vi "date to day of the week.vi"(8 "error in (no error)":errorcluster, 9 "Day":u32, 10 "Month":T2, 11 "Year":u32) -> (0 "error out":errorcluster, 1 "no. of full weeks since 1 Jan 1900":u32, 2 "no. of days since 1 Jan 1900":u32, 3 "Day of the week":T1)   [LabVIEW 2021, in "Project Euler.lvlib"]
uses:
  Project Euler.lvlib
  months_of_the_year enum.ctl
  days_of_the_week enum.ctl
panel:
  out "no. of days in full months in current year":u32
  out "no. of days in current year":u32
  out "full years since 1 Jan 1900":u32[](array[numeric])
  out "no. of days in full years since 1 Jan 1900":u32
  out "no. of full years since 1 Jan 1900":u32
  # "Development\ncontrols/indicators useful for development and testing, but which are not outputs of the VI"
  # "Input\nInputs to the VI"
  # "Output\nOutputs of the VI"
  # "Description\n\nBlank VI with error handling case. \n\nSummarize the use of this VI in this space."
  # "This VI passed this test vector:\nsource = Windows 10 calendar\n1 Jan 1920 = Thursday\n1 Jan 1921 = Saturday\n27 May 1966 = Friday\n30 June 1966 = Thursday\n3 May 1992 = Sunday"
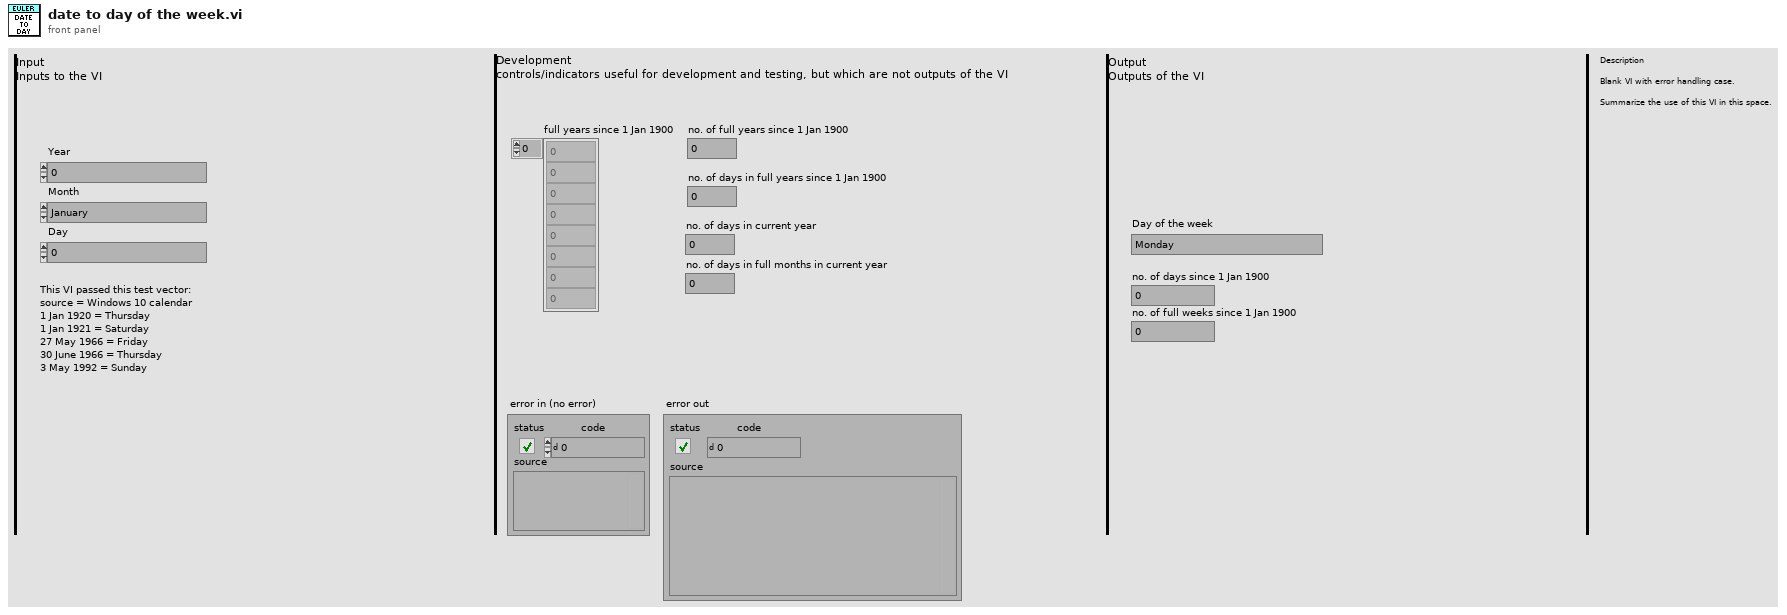
[diagram p1: front panel]
types:
  T1 = typedef "Project Euler.lvlib/days_of_the_week enum.ctl" = enum16{"Monday", "Tuesday", "Wednesday", "Thursday", "Friday", "Saturday", "Sunday"}
  T2 = typedef "Project Euler.lvlib/months_of_the_year enum.ctl" = enum16{"January", "February", "March", "April", "May", "June", "July", "August", "September", "October", "November", "December"}
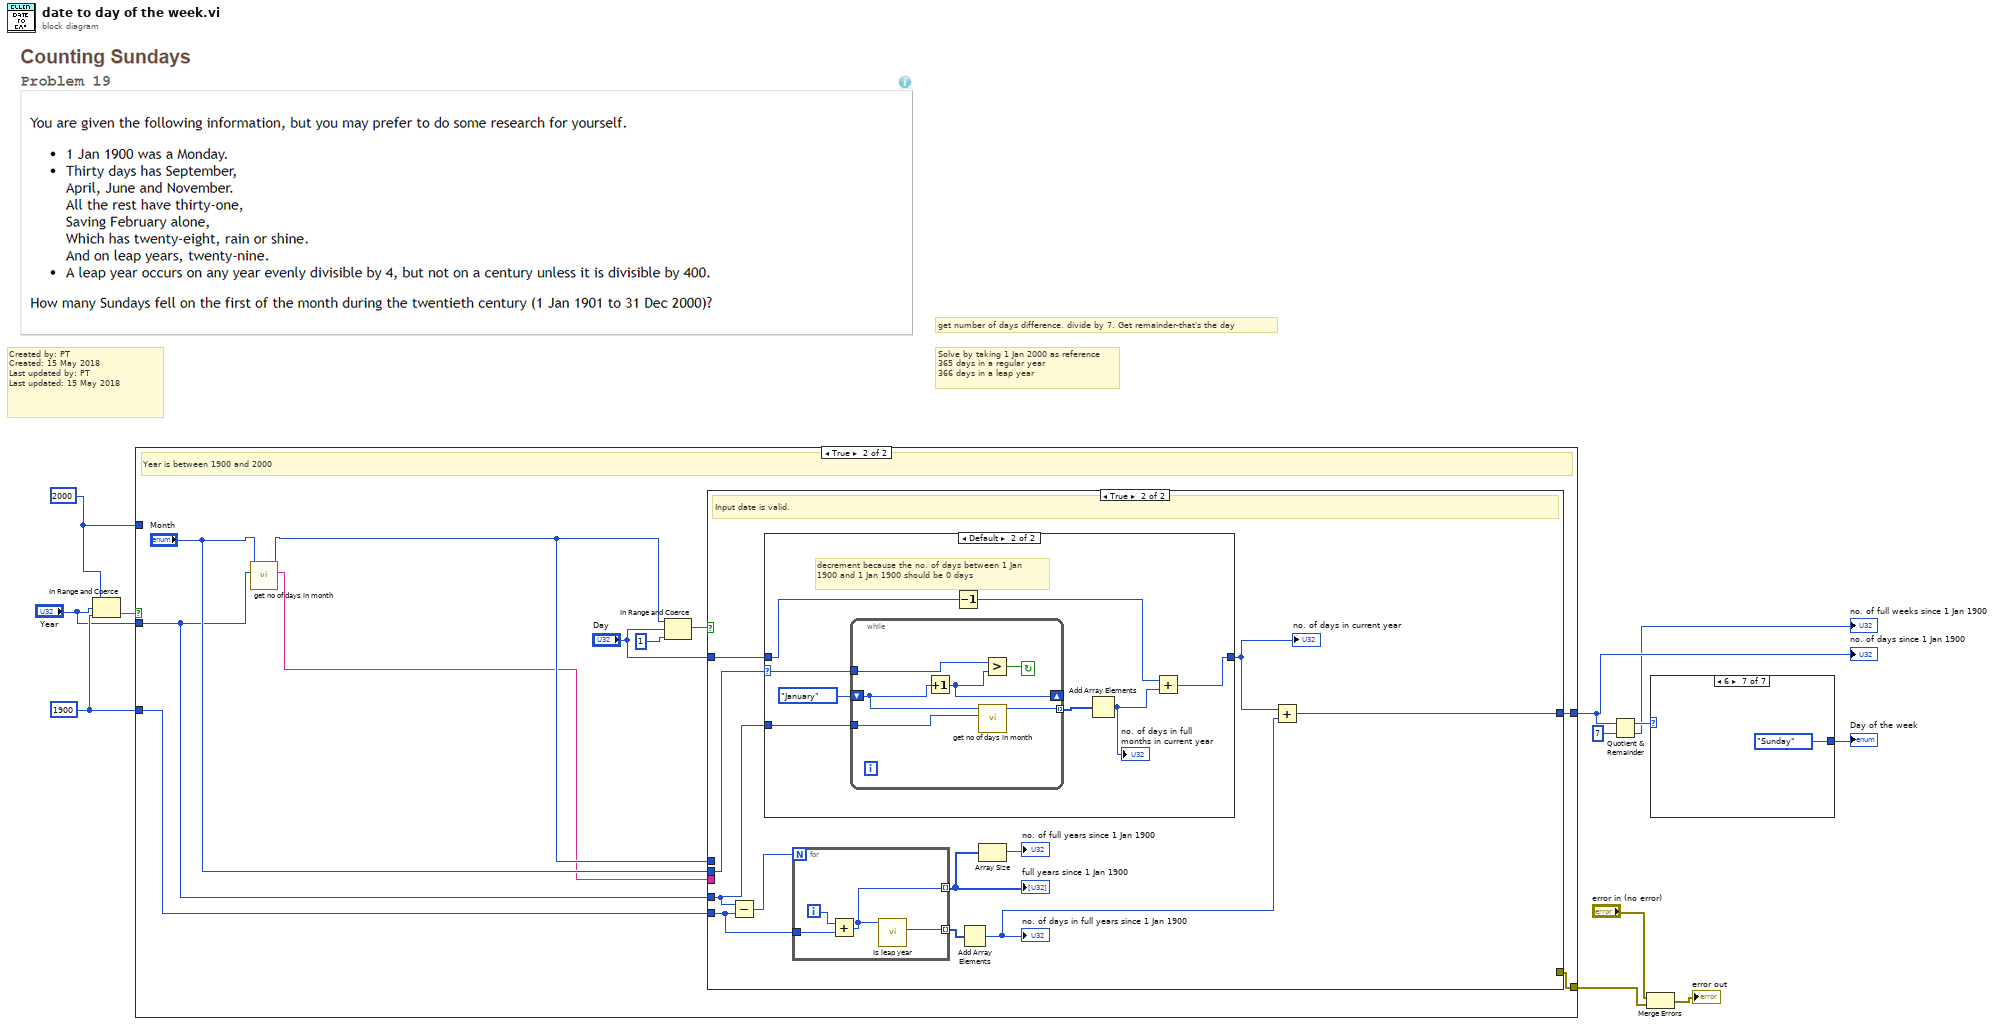
[diagram p0: block diagram]
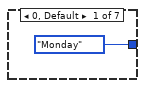
[diagram p2: hidden frame]
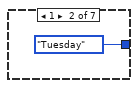
[diagram p3: hidden frame]
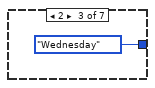
[diagram p4: hidden frame]
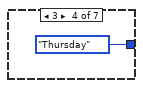
[diagram p5: hidden frame]
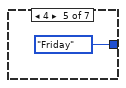
[diagram p6: hidden frame]
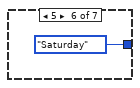
[diagram p7: hidden frame]
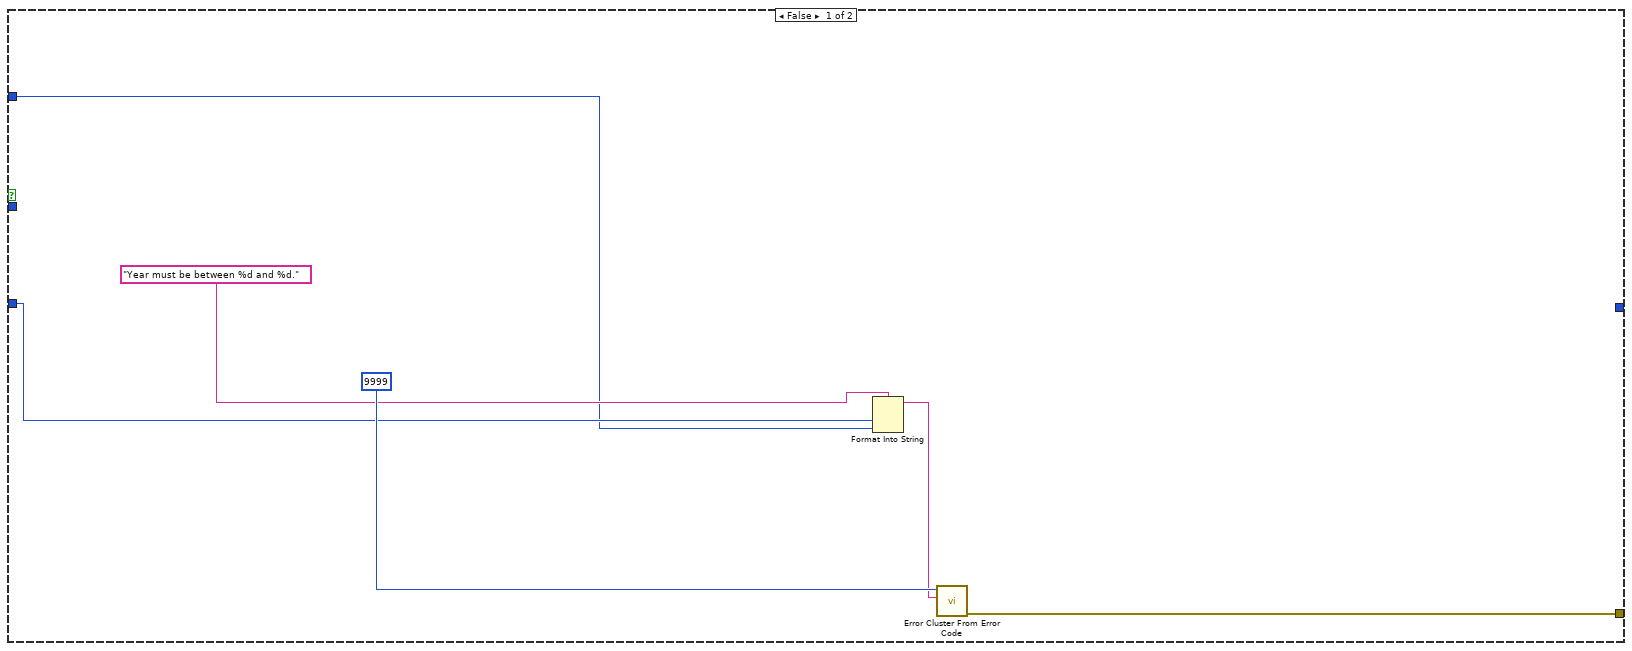
[diagram p8: hidden frame]
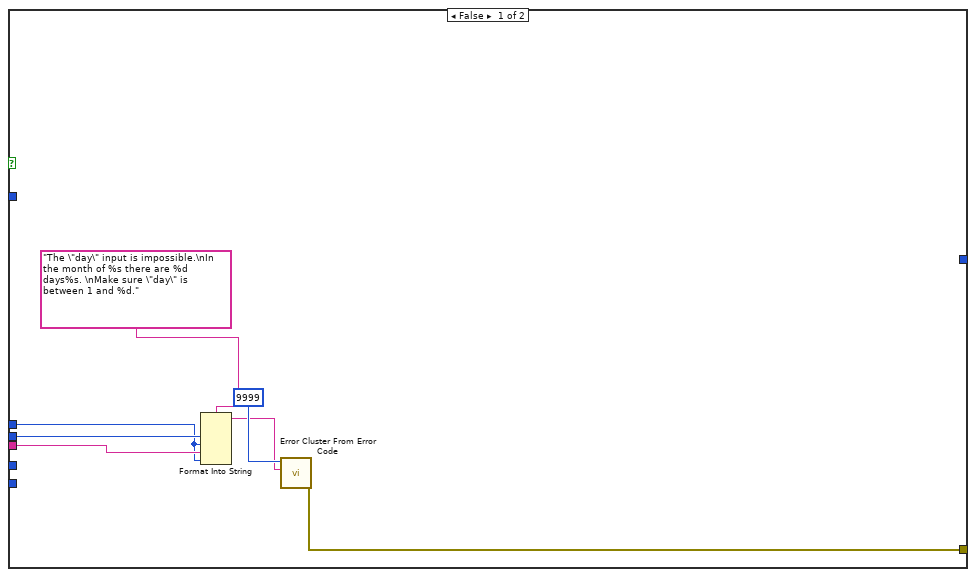
[diagram p9: hidden frame]
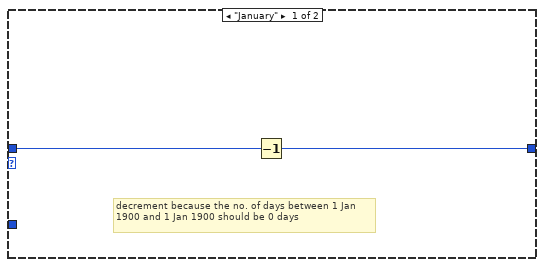
[diagram p10: hidden frame]
diagram:
  w9 = u32 2000 ("lower limit")
  w10 = u32 1900 ("lower limit")
  # "get number of days difference. divide by 7. Get remainder-that's the day"
  # "Solve by taking 1 Jan 2000 as reference\n365 days in a regular year\n366 days in a leap year"
  # "Created by: PT\nCreated: 15 May 2018\nLast updated by: PT\nLast updated: 15 May 2018"
  n1 = In Range and Coerce(upper limit=w9, x="Year", lower limit=w10) -> (In Range?=w11:bool)  [unwired: 1 out]
  n2 = case shown="True" w11 {
    tunnel: [w18 w26] -> w6
    tunnel: w10 -> [w14 w25]
    tunnel: w9 -> [w13 _]
    tunnel: "Year" -> [_ w22]
    tunnel: [_ w19] -> w5
    frame False {
      n3 = Format Into String(format string="Year must be between %d and %d." ("error message (\"\")"), w14, w13) -> (resulting string=w15:string)  [unwired: 2 in, 1 out]
      n4 = call <vilib>:"Error Cluster From Error Code.vi"("error message (\"\")"=w15, "error code (0)"=9999) -> ("error out"=w18:errorcluster)  [unwired: 7 in]
    }
    frame True {
      # "Year is between 1900 and 2000"
      n5 = call "get no of days in month.vi"("Year"=w22, "Month"="Month") -> ("info message"=w20:string, "no. of days this month"=w21:u32)  [unwired: 7 in, 1 out]
      n6 = In Range and Coerce(upper limit=w21, x="Day", lower limit=u32 1) -> (In Range?=w27:bool)  [unwired: 1 out]
      n7 = case shown="True" w27 {
        tunnel: [w35 _] -> w26
        tunnel: "Month" -> [w31 w37]
        tunnel: w21 -> [w29 _]
        tunnel: w20 -> [w30 _]
        tunnel: w22 -> [_ w40]
        tunnel: w25 -> [_ w45]
        tunnel: "Day" -> [_ w41]
        tunnel: [_ w36] -> w19
        frame False {
          n8 = Format Into String(format string="The \"day\" input is impossible.\nIn the month of %s there are %d days%s. \nMake sure \"day\" is between 1 and %d.", w31, w29, w30, w29) -> (resulting string=w32:string)  [unwired: 2 in, 1 out]
          n9 = call <vilib>:"Error Cluster From Error Code.vi"("error message (\"\")"=w32, "error code (0)"=9999) -> ("error out"=w35:errorcluster)  [unwired: 7 in]
        }
        frame True {
          # "Input date is valid."
          n10 = Subtract(x=w40, y=w45) -> (x-y=w46:u32)
          n11 = case shown="Default" w37 {
            selector: w37 -> [_ w56]
            tunnel: w41 -> [w48 w53]
            tunnel: [w47 w50] -> w39
            tunnel: w40 -> [_ w54]
            frame "January" {
              # "decrement because the no. of days between 1 Jan 1900 and 1 Jan 1900 should be 0 days"
              n12 = Decrement(x=w48) -> (x-1=w47:u32)
            }
            frame Default {
              # "decrement because the no. of days between 1 Jan 1900 and 1 Jan 1900 should be 0 days"
              n13 = while {
                tunnel: w56 -> [w62]
                shift-right: [w57] -> _
                shift-left: months_of_the_year_enum."January" ("month") -> [w58]
                tunnel: w54 -> [w60]
                tunnel: [w59] -> w52 mode=indexing
                stop <- w61 continue-if-true
                n14 = Increment(x=w58) -> (x+1=w57:T2)
                n15 = call "get no of days in month.vi"("Year"=w60, "Month"=w58) -> ("no. of days this month"=w59:u32)  [unwired: 7 in, 2 out]
                n16 = Greater?(x=w62, y=w57) -> (0:w61:bool)
              }
              n17 = Decrement(x=w53) -> (x-1=w49:u32)
              n18 = Add Array Elements(numeric array=w52) -> (sum=w51:u32)
              "no. of days in full months in current year" <- w51
              n19 = Add(x=w49, y=w51) -> (x+y=w50:u32)
            }
          }
          "no. of days in current year" <- w39
          n20 = for {
            N: w46 -> [_]
            tunnel: w45 -> [w65]
            tunnel: [w64] -> w44 mode=indexing
            tunnel: [w63] -> w42 mode=indexing
            i -> [w66]
            n21 = Add(x=w66, y=w65) -> (x+y=w63:u32)
            n22 = call "Is leap year.vi"("Year"=w63) -> ("no. of days in year"=w64:u32)  [unwired: 8 in, 2 out]
          }
          "full years since 1 Jan 1900" <- w42
          n23 = Add Array Elements(numeric array=w44) -> (sum=w38:u32)
          "no. of days in full years since 1 Jan 1900" <- w38
          n24 = Array Size(array=w42) -> (size(s)=→"no. of full years since 1 Jan 1900":i32)
          n25 = Add(x=w39, y=w38) -> (x+y=w36:u32)
        }
      }
    }
  }
  "no. of days since 1 Jan 1900" <- w5
  n26 = Quotient & Remainder(x=w5, y=u32 7) -> (x-y*floor(x/y)=w3:u32, floor(x/y)=→"no. of full weeks since 1 Jan 1900":u32)
  n27 = Merge Errors("error in (no error)", w6) -> (→"error out":errorcluster)
  n28 = case shown="6" w3 {
    tunnel: [days_of_the_week_enum."Monday" ("Day of the week") days_of_the_week_enum."Tuesday" ("Day of the week") days_of_the_week_enum."Wednesday" ("Day of the week") days_of_the_week_enum."Thursday" ("Day of the week") days_of_the_week_enum."Friday" ("Day of the week") days_of_the_week_enum."Saturday" ("Day of the week") days_of_the_week_enum."Sunday" ("Day of the week")] -> w2
    frame 0, Default {
    }
    frame 1 {
    }
    frame 2 {
    }
    frame 3 {
    }
    frame 4 {
    }
    frame 5 {
    }
    frame 6 {
    }
  }
  "Day of the week" <- w2
